vi "1NNN.vi"(11 "Variables and Memory in":T1 {"GFX" format="%02x"}) -> (3 "Variables and Memory out":T1 {"GFX" format="%02x"})   [LabVIEW 2021]
uses:
  Controls/ClusterF.ctl
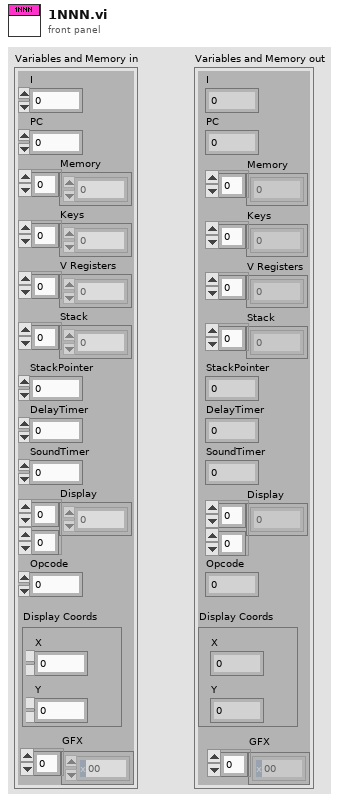
[diagram p1: front panel]
types:
  T1 = typedef "ClusterF.ctl" = cluster{"I":u16, "PC":u16, "Memory":u8[], "Keys":u8[], "V Registers":u8[], "Stack":u16[], "StackPointer":u16, "DelayTimer":u8, "SoundTimer":u8, "Display":u8[][], "Opcode":u16, "Display Coords":cluster{"X":u8, "Y":u8}, "GFX":u8[]}
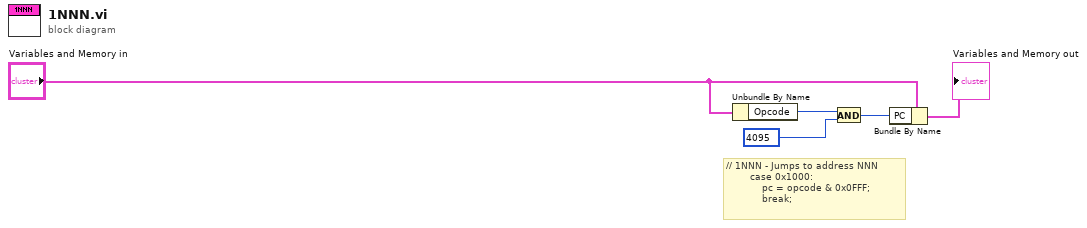
[diagram p0: block diagram]
diagram:
  # "// 1NNN - Jumps to address NNN\n        case 0x1000:\n            pc = opcode & 0x0FFF;\n            break;"
  n1 = Unbundle By Name("Variables and Memory in") -> ("Opcode"=w1:u16)
  n2 = And(x=w1, y=u16 4095) -> (x .and. y?=w5:u16)
  n3 = Bundle By Name(cluster="Variables and Memory in", "PC"=w5) -> (→"Variables and Memory out":T1)
